vi "Agilent 3458 Acquire Single Measurement.vi"() -> ()   [LabVIEW 2020, in "3458A Basic Driver.lvlib"]
doc: "Shows how to configure a measurement and take a reading."
uses:
  3458A Basic Driver.lvlib
  Public/Data/Read Measurement(Single Point).vi
panel:
  in  "Manual Range (1.00)":dbl=1.0 format="%_3g"
  out "Measurement":dbl
  in  "Auto Range (1:ON)":u16(ring)=1 items=["OFF", "ON", "ONCE"]
  in  "Frequency Source (3: AC Voltage)":u16(ring)=3 items=["AC + DC Current", "AC + DC Voltage", "AC Current", "AC Voltage"]
  in  "Trigger Type (0:Auto)":u16(ring) items=["Auto", "External", "Level", "Line", "Synchronous"]
  in  "Manual Resolution (2: 6.5 digits)":enum16{"4.5", "5.5", "6.5", "7.5", "8.5"}(ring)=enum."6.5"
  in  "Function (0: DC Voltage)":u16(ring) items=["DC Voltage", "AC Voltage", "AC + DC Voltage", "DC Current", "AC Current", "AC + DC Current", "2-Wire Resistance", "4-Wire Resistance", "Frequency", "Period", "Direct Sampling DC", "Direct Sampling AC"]
  in  "VISA resource name":refnum<visa-resource-name>
  # "(c) 2007  National Instruments.  ALL RIGHTS RESERVED."
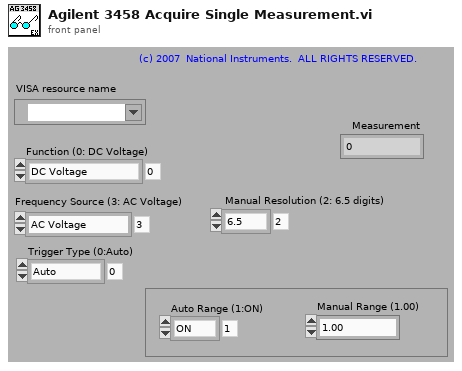
[diagram p1: front panel]
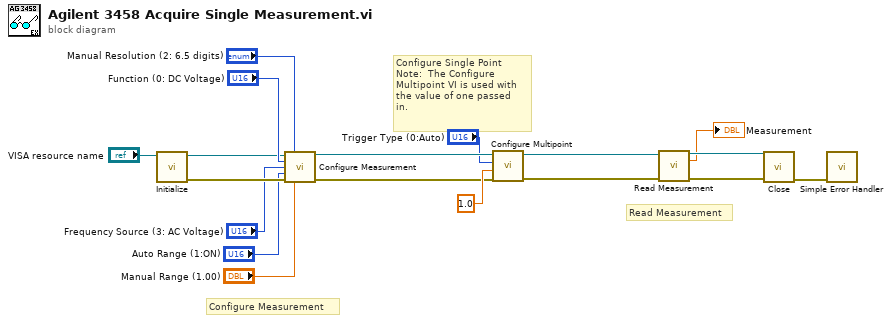
[diagram p0: block diagram]
diagram:
  # "Configure Single Point\nNote:  The Configure \nMultipoint VI is used with\nthe value of one passed\nin."
  # "Read Measurement"
  # "Configure Measurement"
  n1 = call "Initialize.vi"("VISA resource name"="VISA resource name") -> ("error out"=w8:errorcluster, "VISA resource name out"=w9:refnum<visa-resource-name>)  [unwired: 8 in, 1 out]
  n2 = call "Configure Measurement.vi"("VISA resource name"=w9, "Manual Resolution (2: 6.5 digits)"="Manual Resolution (2: 6.5 digits)", "Function (0: DC Voltage)"="Function (0: DC Voltage)", "Frequency Source (3: AC Voltage)"="Frequency Source (3: AC Voltage)", "Auto Range (1:ON)"="Auto Range (1:ON)", "error in (no error)"=w8, "Manual Range (1.00)"="Manual Range (1.00)") -> ("VISA resource name out"=w12:refnum<visa-resource-name>, "error out"=w11:errorcluster)  [unwired: 7 in]
  n3 = call "Configure Multipoint.vi"("error in (no error)"=w11, "Sample Count (1)"=1.0, "Trigger Type (0:Auto)"="Trigger Type (0:Auto)", "VISA resource name"=w12) -> ("error out"=w6:errorcluster, "VISA resource name out"=w7:refnum<visa-resource-name>)  [unwired: 6 in]
  n4 = call-poly "Read Measurement.vi"("VISA resource name"=w7, "error in (no error)"=w6) -> ("VISA resource name out"=w15:refnum<visa-resource-name>, "Measurement"=→"Measurement":dbl, "error out"=w14:errorcluster)  [unwired: 11 in]
  n5 = call "Close.vi"("error in (no error)"=w14, "VISA resource name"=w15) -> ("error out"=w13:errorcluster)  [unwired: 9 in]
  n6 = call <vilib>:"Simple Error Handler.vi"("error in (no error)"=w13) -> ()  [unwired: 4 in, 5 out]
